vi "EditSettings.vi"(11 "Template in":string) -> (1 "Settings out":T1={"Name of test"="", "Date"=timestamp(0 s since 1904-01-01), "Location"="", "Template"="", "Soundcard"="", "resolution"=32, "Sampling rate"=48000, "Ch1 Gain "=25.0, "Ch2 Gain"=10.0, "Sample time (s)"=0.3, "Pre-trigger (s)"=0.01, "Hammer Threshold"=10.0, "Positions"=12, "Taps/Position"=5, "Set Names"="", "Freq resolution"=10.0, "Hammer cutoff"=0.0, "Mic cutoff"=0.0, "Double bounce "=0.0, "Hammer Cal"=1.0, "dB Offset"=0.0, "Accel Cal"=1.0, "Vibrometer Cal"=1.0, "Mic Cal"=1.0, "Output"=2, "Voltage Cal"=1.0, "Vibrometer Port"="ASRL27::INSTR", "Range"=50, "High Pass"=2, "Bandwidth"=25, "X Range"=[], "Y Range"=[], "dB Spread"=0.0, "Trigger"=0, "Ch_1"=1, "Ch_2"=2, "flip?"=FALSE, "60Hz"=FALSE, "Time offset"=0.0, "Piezo Cal"=1.0, "Default Notes"="", "Tom"=FALSE} {"Ch_2" min=1 step=1; "Ch_1" min=1 max=100 step=1; "Trigger" items=["Hammer (force)", "Self-tap", "Spacebar"]; "Bandwidth" items=["1 kHz"=1, "5 kHz"=5, "10 kHz"=10, "25 kHz"=25, "50 kHz"=50, "100 kHz"=100]; "High Pass" items=["Off", "13 Hz", "104 Hz"]; "Range" items=["10 mm/s"=1, "20 mm/s"=2, "50 mm/s"=5, "100 mm/s"=10, "200 mm/s"=20, "500 mm/s"=50, "1 m/s"=100, "2 m/s"=200]; "Output" items=["Accelerometer", "Speed (from acceleration)", "Microphone", "Vibrometer", "Piezo"]; "Voltage Cal" format="%#_13g"; "Ch2 Gain" format="%#_13g"; "Ch1 Gain" format="%#_13g"; "Double bounce" min=0.0; "Mic cutoff" min=0.0 format="%#_4g"; "Hammer cutoff" min=0.0 format="%#_4g"; "Freq resolution" min=0.0; "Pre-trigger (s)" format="%#_13g"; "Date" format="%<%H:%M\n%d/%m/%y>T"; "resolution" items=["16 bit"=16, "24 bit"=24, "32 bit"=32]; "Sampling rate" items=["22050 samp/s"=22050, "44100 samp/s"=44100, "48000 samp/s"=48000]}, 3 "Template out":string)   [LabVIEW 2022 SP3]
uses:
  Mic/Mic_Global.vi
  PreferencesControl.ctl
panel:
  in  "Import Cal":bool
  in  "Advanced":bool
  out "Hammer Spectrum":cluster{dbl, "df":dbl, "FFT {X}":dbl[]}[](graph)=[{0.0, "df"=1.0, "FFT {X}"=array[24000 elements]}, {0.0, "df"=40000.0, "FFT {X}"=[-20.0, -20.0]}]
  in  "Vibrometer":bool
  in  "delete":bool
  in  "Update":bool
  in  "Template":u16(ring) items=["Admittance H modified", "Admittance H", "Admittance Scratchpad", "JC H 12 radiation", "JC H 7 radiation modified modified", "JC H 7 radiation modified", "JC H 7 radiation", "JC HV 24 radiation", "Radiation ScratchPad", "ScratchPad", "TapTones ScratchPad", "TEST modified", "TEST"]
  in  "Graph Ranges":T2={"Ranges"=[{"XMin"=200.0, "XMax"=10000.0, "XInc"=2500.0, "XMinor"=500.0, "YMin"=-25.0, "YMax"=0.0, "YInc"=5.0, "YMinor"=1.0}, {"XMin"=0.0, "XMax"=0.05, "XInc"=0.025, "XMinor"=0.0025, "YMin"=-0.1, "YMax"=0.1, "YInc"=0.05, "YMinor"=0.01}, {"XMin"=0.0, "XMax"=0.3, "XInc"=0.1, "XMinor"=0.01, "YMin"=-0.1, "YMax"=0.1, "YInc"=0.05, "YMinor"=0.01}, {"XMin"=200.0, "XMax"=10000.0, "XInc"=10.0, "XMinor"=100.0, "YMin"=-30.0, "YMax"=30.0, "YInc"=5.0, "YMinor"=1.0}]}
  in  "Save":bool
  in  "Cancel Button":bool
  in  "Save as a Template":bool
  in  "Import Template":bool
  out "Template file":string
  in  "Settings":T3={"Name of test"="ScratchPad", "Date"=timestamp(0 s since 1904-01-01), "Location"="Home", "Default Template"="", "Soundcard"="OCTA-CAPTURE", "resolution"=32, "Sampling rate"=48000, "Ch1 Gain "=10.0, "Ch2 Gain"=20.0, "Sample time (s)"=0.3, "Pre-trigger (s)"=0.001, "Hammer Threshold"=0.01, "Positions"=12, "Taps/Position"=5, "Set Names"="H,V", "Freq resolution"=1.0, "Hammer cutoff"=0.025, "Mic cutoff"=0.25, "Double bounce "=0.01, "Hammer Cal"=1.0, "dB Offset"=0.0, "Accel Cal"=1.0, "Vibrometer Cal"=1.0, "Mic Cal"=49.38, "Output"=2, "Voltage Cal"=13.8, "Vibrometer Port"="ASRL27::INSTR", "Range"=50, "High Pass"=2, "Bandwidth"=25, "X Range"=[{"Minimum"=200.0, "Maximum"=10000.0, "Increment"=2500.0, "Minor Increment"=500.0, "Start"=2500.0}, {"Minimum"=0.0, "Maximum"=0.05, "Increment"=0.025, "Minor Increment"=0.0025, "Start"=0.0}, {"Minimum"=0.0, "Maximum"=0.3, "Increment"=0.1, "Minor Increment"=0.01, "Start"=0.0}, {"Minimum"=200.0, "Maximum"=10000.0, "Increment"=10.0, "Minor Increment"=100.0, "Start"=1000.0}], "Y Range"=[{"Minimum"=-25.0, "Maximum"=0.0, "Increment"=5.0, "Minor Increment"=1.0, "Start"=-25.0}, {"Minimum"=-0.1, "Maximum"=0.1, "Increment"=0.05, "Minor Increment"=0.01, "Start"=-0.1}, {"Minimum"=-0.1, "Maximum"=0.1, "Increment"=0.05, "Minor Increment"=0.01, "Start"=-0.1}, {"Minimum"=-30.0, "Maximum"=30.0, "Increment"=5.0, "Minor Increment"=1.0, "Start"=-30.0}], "dB Spread"=40.0, "Trigger"=0, "Ch_1"=1, "Ch_2"=2, "flip?"=FALSE, "60Hz"=FALSE, "Time Offset"=1.0, "Piezo Cal"=1.0, "Default Notes for template"="H,V", "Tom"=FALSE} {"Voltage Cal" format="%#_13g"; "Freq resolution" min=0.0; "Pre-trigger (s)" format="%#_13g"; "resolution" items=["16 bit"=16, "24 bit"=24, "32 bit"=32]; "Sampling rate" items=["22050 samp/s"=22050, "44100 samp/s"=44100, "48000 samp/s"=48000]; "Ch_2" min=1 step=1; "Ch_1" min=1 max=100 step=1; "Trigger" items=["Hammer (force)", "Self-tap", "Spacebar"]; "Bandwidth" items=["1 kHz"=1, "5 kHz"=5, "10 kHz"=10, "25 kHz"=25, "50 kHz"=50, "100 kHz"=100]; "High Pass" items=["Off", "13 Hz", "104 Hz"]; "Range" items=["10 mm/s"=1, "20 mm/s"=2, "50 mm/s"=5, "100 mm/s"=10, "200 mm/s"=20, "500 mm/s"=50, "1 m/s"=100, "2 m/s"=200]; "Output" items=["Accelerometer", "Speed (accelerometer)", "Microphone", "Vibrometer"]; "Ch2 Gain" format="%#_13g"; "Ch1 Gain" format="%#_13g"; "Double bounce" min=0.0; "Mic cutoff" min=0.0 format="%#_4g"; "Hammer cutoff" min=0.0 format="%#_4g"; "Date" format="%<%H:%M\n%d/%m/%y>T"}
  out "Hammer Data":cluster{dbl, "dt":dbl, "Y":dbl[]}[](graph)=[{0.0, "dt"=2.0833333333333333e-05, "Y"=array[14400 elements]}, {0.0, "dt"=0.0, "Y"=[]}]
  out "Microphone Data":cluster{dbl, "dt":dbl, "Y":dbl[]}[](graph)=[{0.0, "dt"=2.0833333333333333e-05, "Y"=array[14400 elements]}, {0.0, "dt"=0.0, "Y"=[]}]
  out "Average FRF":cluster{dbl, "df":dbl, dbl[]}[](graph)=[{0.0, "df"=1.0, array[24000 elements]}, {0.0, "df"=1.0, array[24000 elements]}]
  # "Adjust default scale ranges"
  # "Hz"
  # "dB"
  # "dB"
  # "sec"
  # "sec"
  # "mV/Pa"
  # "mV/m/s2"
  # "mV/mm/s"
  # "V/N"
  # "sec"
  # "sec"
  # "mV/N"
  # "a.u."
  # "a.u."
  # "sec"
  # "X Min      X Max      X Inc        X Minor   Y Min      Y Max       Y Inc        Y Minor"
  # "Hammer Spectrum\n\nHammer Level Meter \n\nMic Level Meter\n\nFreq Response Plot"
  # "mV/Pa"
  # "mV/m/s2"
  # "mV/mm/s"
  # "Hz"
  # "V/N"
  # "dB"
  # "sec"
  # "sec"
  # "dB"
  # "mV/N"
  # "a.u."
  # "sec"
  # "a.u."
  # "sec"
  # "sec"
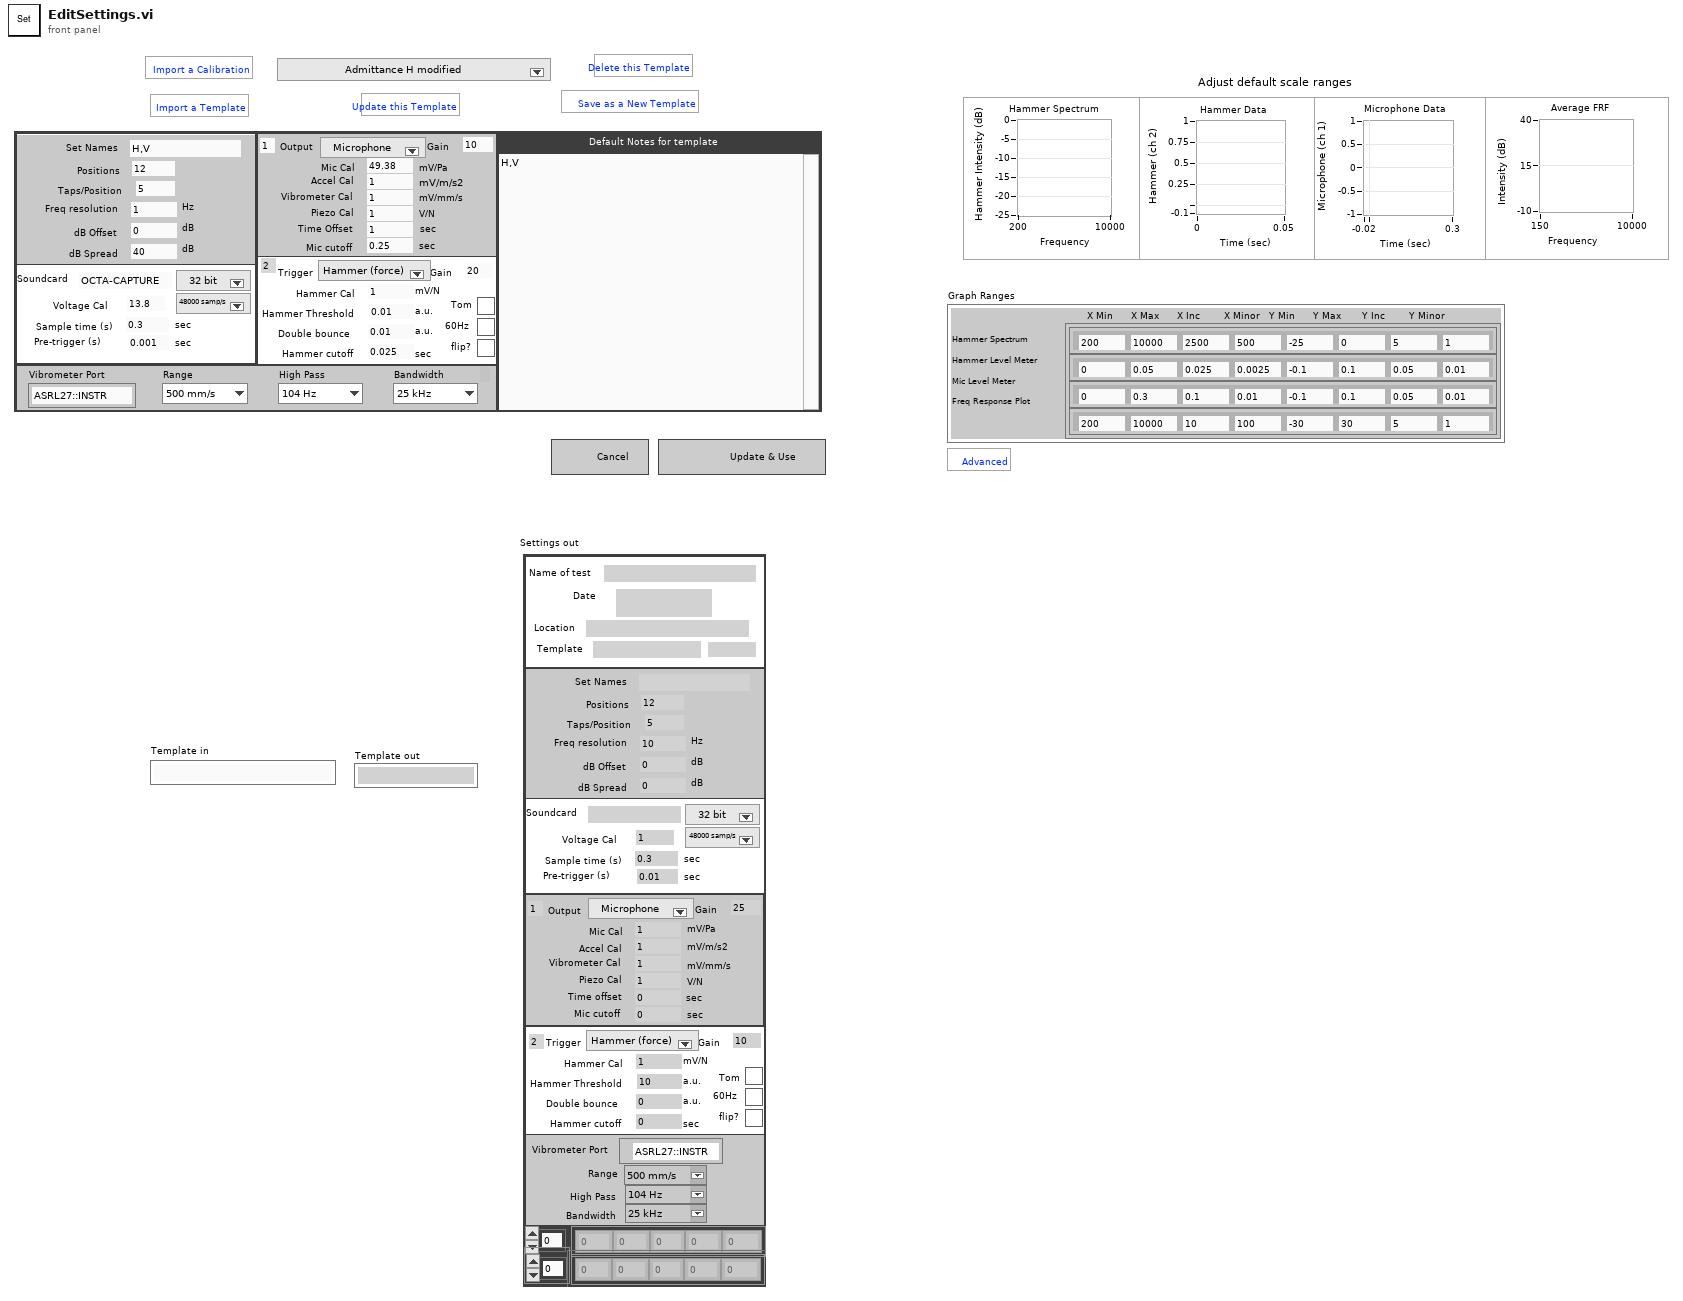
[diagram p1: front panel]
types:
  T1 = typedef "PreferencesControl.ctl" = cluster{"Name of test":string, "Date":timestamp, "Location":string, "Template":string, "Soundcard":string, "resolution":u16, "Sampling rate":u16, "Ch1 Gain ":dbl, "Ch2 Gain":dbl, "Sample time (s)":dbl, "Pre-trigger (s)":dbl, "Hammer Threshold":dbl, "Positions":i16, "Taps/Position":i16, "Set Names":string, "Freq resolution":dbl, "Hammer cutoff":dbl, "Mic cutoff":dbl, "Double bounce ":dbl, "Hammer Cal":dbl, "dB Offset":dbl, "Accel Cal":dbl, "Vibrometer Cal":dbl, "Mic Cal":dbl, "Output":u16, "Voltage Cal":dbl, "Vibrometer Port":refnum<visa-resource-name>, "Range":u16, "High Pass":u16, "Bandwidth":u16, "X Range":cluster{"Minimum":dbl, "Maximum":dbl, "Increment":dbl, "Minor Increment":dbl, "Start":dbl}[], "Y Range":cluster{"Minimum":dbl, "Maximum":dbl, "Increment":dbl, "Minor Increment":dbl, "Start":dbl}[], "dB Spread":dbl, "Trigger":u16, "Ch_1":u8, "Ch_2":u8, "flip?":bool, "60Hz":bool, "Time offset":dbl, "Piezo Cal":dbl, "Default Notes":string, "Tom":bool}
  T2 = cluster{"Ranges":cluster{"XMin":dbl, "XMax":dbl, "XInc":dbl, "XMinor":dbl, "YMin":dbl, "YMax":dbl, "YInc":dbl, "YMinor":dbl}[]}
  T3 = cluster{"Name of test":string, "Date":timestamp, "Location":string, "Default Template":string, "Soundcard":string, "resolution":u16, "Sampling rate":u16, "Ch1 Gain ":dbl, "Ch2 Gain":dbl, "Sample time (s)":dbl, "Pre-trigger (s)":dbl, "Hammer Threshold":dbl, "Positions":i16, "Taps/Position":i16, "Set Names":string, "Freq resolution":dbl, "Hammer cutoff":dbl, "Mic cutoff":dbl, "Double bounce ":dbl, "Hammer Cal":dbl, "dB Offset":dbl, "Accel Cal":dbl, "Vibrometer Cal":dbl, "Mic Cal":dbl, "Output":u16, "Voltage Cal":dbl, "Vibrometer Port":string, "Range":u16, "High Pass":u16, "Bandwidth":u16, "X Range":cluster{"Minimum":dbl, "Maximum":dbl, "Increment":dbl, "Minor Increment":dbl, "Start":dbl}[], "Y Range":cluster{"Minimum":dbl, "Maximum":dbl, "Increment":dbl, "Minor Increment":dbl, "Start":dbl}[], "dB Spread":dbl, "Trigger":u16, "Ch_1":u8, "Ch_2":u8, "flip?":bool, "60Hz":bool, "Time Offset":dbl, "Piezo Cal":dbl, "Default Notes for template":string, "Tom":bool}
  T4 = enum8{"Enabled", "Disabled", "Disabled and Grayed Out"}
  T5 = enum32{"Invalid", "Default", "Floating", "Floating/Auto-Hide", "Modal"}
  T6 = typedef "LVRangeTypeDef.ctl" = cluster{"Minimum":dbl, "Maximum":dbl, "Increment":dbl, "Minor Increment":dbl, "Start":dbl}
  T7 = typedef "LVRectTypeDef.ctl" = cluster{"Left":i16, "Top":i16, "Right":i16, "Bottom":i16}
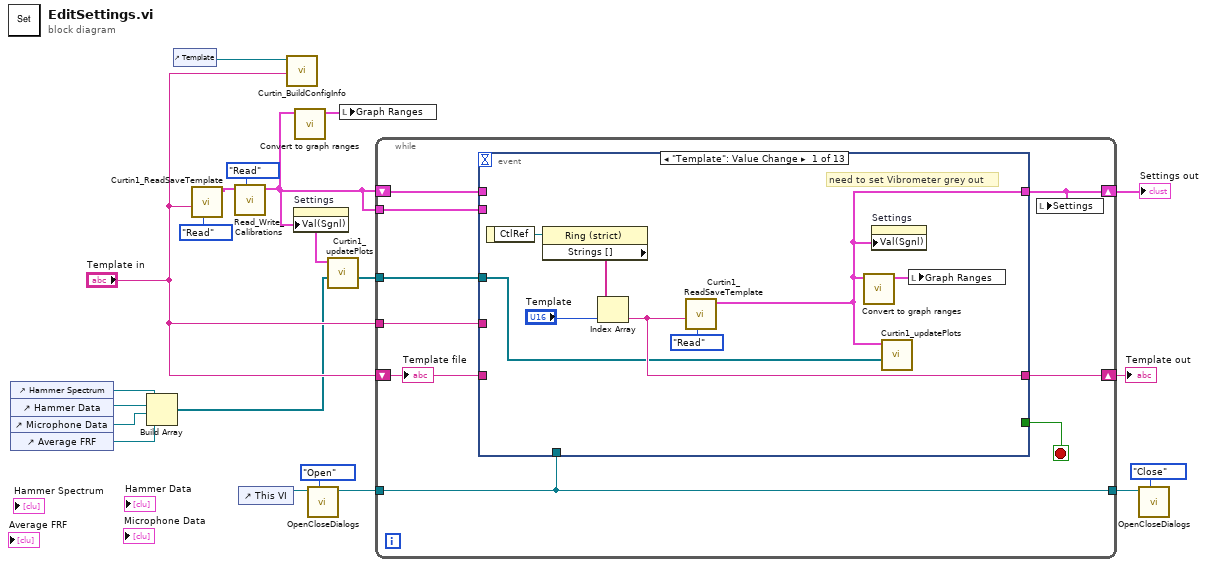
[diagram p0: block diagram]
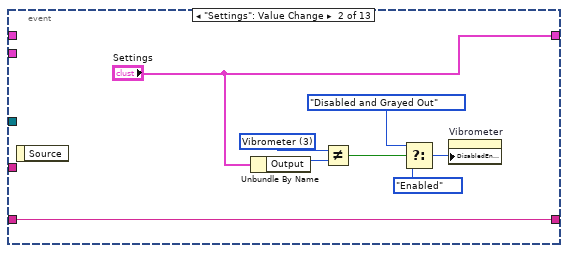
[diagram p2: hidden frame]
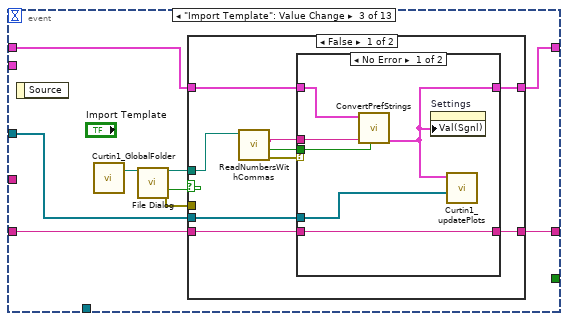
[diagram p3: hidden frame]
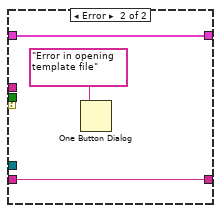
[diagram p4: hidden frame]
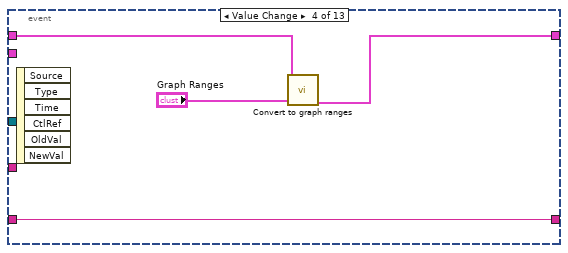
[diagram p6: hidden frame]
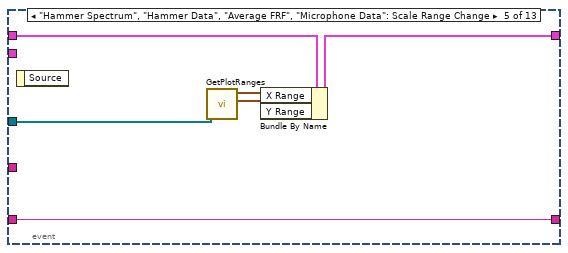
[diagram p7: hidden frame]
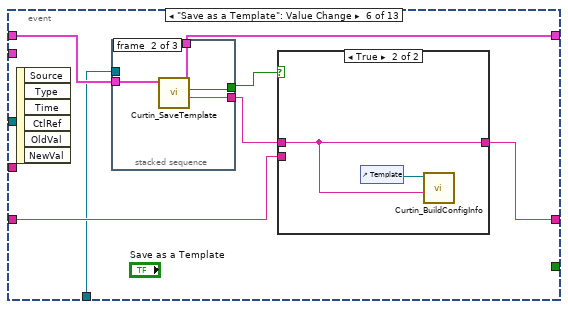
[diagram p8: hidden frame]
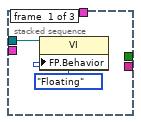
[diagram p9: hidden frame]
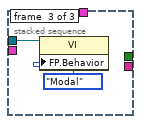
[diagram p10: hidden frame]
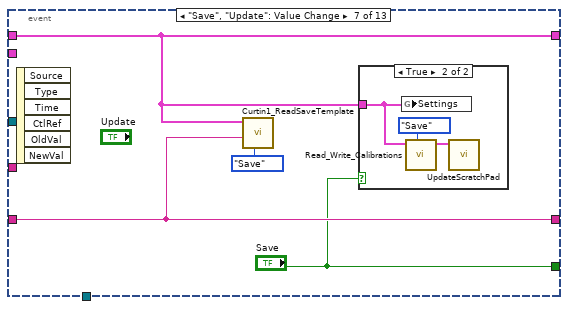
[diagram p12: hidden frame]
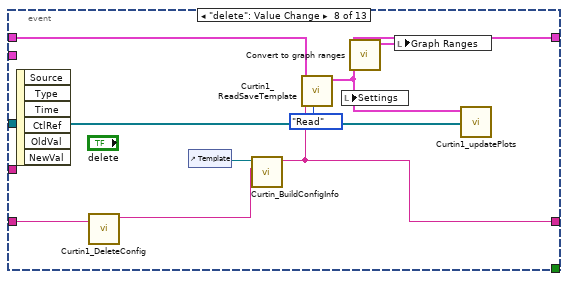
[diagram p14: hidden frame]
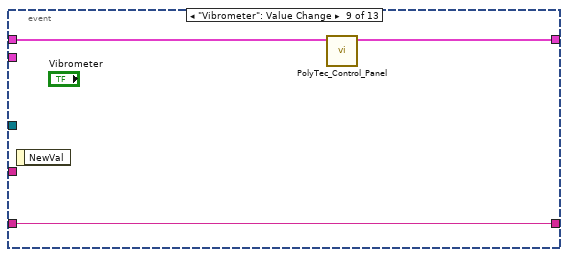
[diagram p15: hidden frame]
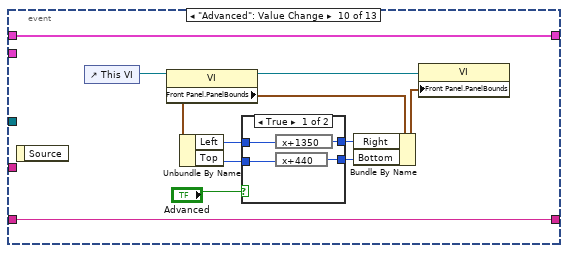
[diagram p16: hidden frame]
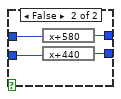
[diagram p17: hidden frame]
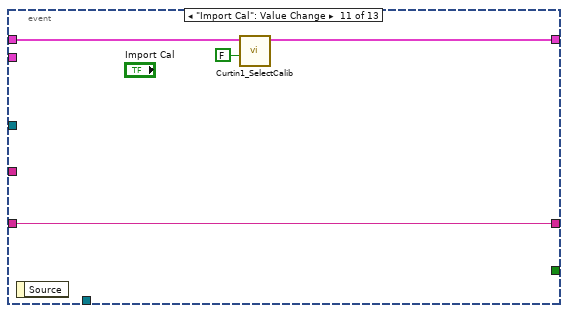
[diagram p18: hidden frame]
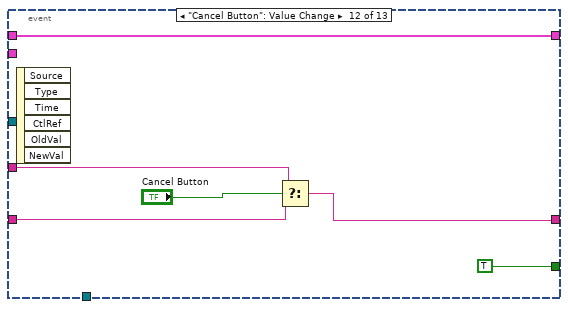
[diagram p19: hidden frame]
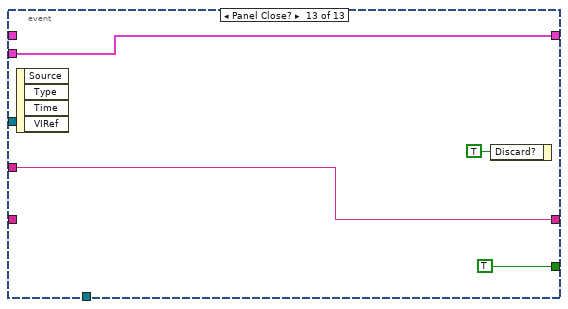
[diagram p20: hidden frame]
diagram:
  n1 = control-ref of="Hammer Spectrum"() -> (w11:refnum<vi>)
  n2 = control-ref of="Hammer Data"() -> (w12:refnum<vi>)
  n3 = control-ref of="Microphone Data"() -> (w13:refnum<vi>)
  n4 = control-ref of="Average FRF"() -> (w14:refnum<vi>)
  n5 = Build Array(w11, w12, w13, w14) -> (w10:refnum<vi>[])
  n6 = control-ref of="Template"() -> (w16:refnum<vi>)
  n7 = call "Curtin1_ReadSaveTemplate.vi"("Task"=enum16{"Save", "Read", "List"}."Read", "Template"="Template in") -> ("Settings out"=w7:T1)  [unwired: 6 in, 3 out]
  n8 = call "Read_Write_Calibrations.vi"("Task"=enum16{"Save", "Read", "List"}."Read", "Settings in"=w7) -> ("Settings out"=w6:T1)  [unwired: 7 in, 2 out]
  n9 = control-ref of="This VI"() -> (w4:refnum<vi>)
  n10 = call "Curtin_BuildConfigInfo.vi"("Test Template in"="Template in", "ComboBox in"=w16) -> ()  [unwired: 8 in, 2 out]
  n11 = property on="Settings" class="Clust (strict)"("Val(Sgnl)"=w6) -> ()  [unwired: 2 in, 2 out]
  n12 = call "Convert to graph ranges.vi"("Settings in"=w6) -> ("Graph Ranges out"=w17:T2)  [unwired: 9 in, 1 out]
  n13 = call "OpenCloseDialogs.vi"("Task"=enum16{"Open", "Close"}."Open", "VI in"=w4) -> ("VI out"=w1:refnum<vi>)  [unwired: 8 in, 1 out]
  n14 = call "Curtin1_updatePlots.vi"("plots"=w10, "Settings"=w6) -> ()  [unwired: 10 in]
  n15 = local write "Graph Ranges"(w17) -> ()
  n16 = while {
    shift-right: [w23] -> w9
    shift-left: w6 -> [w27]
    shift-right: [w26] -> w18
    shift-left: "Template in" -> [w25]
    tunnel: "Template in" -> [w24]
    tunnel: w6 -> [w22]
    tunnel: w10 -> [w21]
    tunnel: [w20] -> w2
    tunnel: w1 -> [w20]
    stop <- w28 stop-if-true
    n17 = event shown="[0] \"Template\": Value Change" {
      selector: _ -> [_ _ _ _ _ _ _ _ _ _ _ _ _]
      dyn-events: _ -> [_ _ _ _ _ _ _ _ _ _ _ _ _]
      timeout: _ -> [_ _ _ _ _ _ _ _ _ _ _ _ _]
      tunnel: [_ _ _ _ _ _ "Save" _ _ _ _ TRUE TRUE] -> w28
      tunnel: w27 -> [_ _ w51 w75 w80 w88 w102 w113 w119 w131 w142 w148 _]
      tunnel: [w29 "Settings" w50 w74 w79 w86 w102 w109 w118 w131 w141 w148 w150] -> w23
      tunnel: [w31 w44 w49 w77 w78 w90 w104 w112 w120 w121 w143 w144 w151] -> w26
      tunnel: w25 -> [_ w44 w48 w77 w78 w89 w104 w117 w120 w121 w143 w145 _]
      tunnel: w24 -> [_ _ _ _ _ _ _ _ _ _ _ w146 w151]
      tunnel: w22 -> [_ _ _ _ _ _ _ _ _ _ _ _ w150]
      tunnel: w21 -> [w30 _ w45 _ w81 _ _ w110 _ _ _ _ _]
      tunnel: w20 -> [_ _ _ _ _ w85 _ _ _ _ _ _ _]
      event "Template": Value Change {
        # "need to set Vibrometer grey out"
        n18 = event-data() -> ("CtlRef"=w34:refnum<vi>)  [unwired: 1 in]
        n19 = property class="Ring (strict)"(reference=w34) -> ("Strings []"=w33:string[])  [unwired: 1 in, 2 out]
        n20 = Index Array(array=w33, index="Template") -> (element=w31:string)
        n21 = call "Curtin1_ReadSaveTemplate.vi"("Task"=enum16{"Save", "Read", "List"}."Read", "Template"=w31) -> ("Settings out"=w29:T1)  [unwired: 6 in, 3 out]
        n22 = call "Convert to graph ranges.vi"("Settings in"=w29) -> ("Graph Ranges out"=w36:T2)  [unwired: 9 in, 1 out]
        n23 = property on="Settings" class="Clust (strict)"("Val(Sgnl)"=w29) -> ()  [unwired: 2 in, 2 out]
        n24 = call "Curtin1_updatePlots.vi"("plots"=w30, "Settings"=w29) -> ()  [unwired: 10 in]
        n25 = local write "Graph Ranges"(w36) -> ()
      }
      event "Settings": Value Change {
        w39 = u16 3 items=["Acclerometer", "Displacement", "Microphone", "Vibrometer"] ("Output")
        n26 = event-data() -> ()  [unwired: 1 in, 1 out]
        n27 = Unbundle By Name("Settings") -> ("Output"=w38:u16)
        n28 = Not Equal?(x=w39, y=w38) -> (x != y?=w40:bool)
        n29 = Select(t=T4."Disabled and Grayed Out" ("Disabled"), s=w40, f=T4."Enabled" ("Disabled")) -> (s? t:f=w43:T4)
        n30 = property on="Vibrometer" class="Bool"("DisabledEnum"=w43) -> ()  [unwired: 2 in, 2 out]
      }
      event "Import Template": Value Change {
        n31 = event-data() -> ()  [unwired: 1 in, 1 out]
        n32 = call "Curtin1_GlobalFolder.vi"() -> ("LabVIEW Data Path"=w46:path)  [unwired: 1 in, 1 out]
        n33 = call "File Dialog"("start path"=w46) -> ("selected path"=w53:path, "cancelled"=w52:bool, "error out"=w47:errorcluster)  [unwired: 11 in, 1 out]
        n34 = case shown="False" w52 {
          tunnel: w53 -> [w57 _]
          tunnel: w51 -> [w62 w73]
          tunnel: [w61 w73] -> w50
          tunnel: [w60 w72] -> w49
          tunnel: w48 -> [w59 w72]
          tunnel: w47 -> [_ _]
          tunnel: w45 -> [w58 _]
          frame False {
            n35 = call "ReadNumbersWithCommas.vi"("file (use dialog)"=w57) -> ("error out"=w55:errorcluster, "comma?"=w54:bool, "text"=w56:string)  [unwired: 7 in, 1 out]
            n36 = case shown="No Error" w55 {
              tunnel: w62 -> [w66 w71]
              tunnel: [w64 w71] -> w61
              tunnel: [w68 w69] -> w60
              tunnel: w59 -> [w68 w69]
              tunnel: w56 -> [w67 _]
              tunnel: w58 -> [w65 _]
              tunnel: w54 -> [w63 _]
              frame No Error {
                n37 = call "ConvertPrefStrings.vi"("Comma?"=w63, "String In"=w67, "Settings"=w66) -> ("Settings"=w64:T1)  [unwired: 7 in, 1 out]
                n38 = property on="Settings" class="Clust (strict)"("Val(Sgnl)"=w64) -> ()  [unwired: 2 in, 2 out]
                n39 = call "Curtin1_updatePlots.vi"("plots"=w65, "Settings"=w64) -> ()  [unwired: 10 in]
              }
              frame Error {
                n40 = One Button Dialog(message="Error in opening template file") -> ()  [unwired: 1 in, 1 out]
              }
            }
          }
          frame True {
          }
        }
      }
      event "Graph Ranges.Ranges": Value Change {
        n41 = event-data() -> ()  [unwired: 1 in, 6 out]
        n42 = call "Convert to graph ranges.vi"("Graph Ranges in"="Graph Ranges", "Settings in"=w75) -> ("Settings out"=w74:T1)  [unwired: 8 in, 1 out]
      }
      event "Hammer Spectrum", "Hammer Data", "Average FRF", "Microphone Data": Scale Range Change {
        n43 = event-data() -> ()  [unwired: 1 in, 1 out]
        n44 = call "GetPlotRanges.vi"("plots"=w81) -> ("Yscales"=w83:T6[], "Xscales"=w82:T6[])  [unwired: 9 in]
        n45 = Bundle By Name(cluster=w80, "X Range"=w82, "Y Range"=w83) -> (w79:T1)
      }
      event "Save as a Template": Value Change {
        n46 = event-data() -> ()  [unwired: 1 in, 6 out]
        n47 = stacked-sequence {
          tunnel: w85 -> [w92 _ w98]
          tunnel: w88 -> [_ w96 _]
          tunnel: [_ w95 _] -> w87
          tunnel: [_ w94 _] -> w84
          tunnel: [_ w93 _] -> w86
          frame #0 {
            n48 = property class="VI"(reference=w92, "FP.Behavior"=T5."Floating" ("Front Panel Window:Behavior")) -> ()  [unwired: 1 in, 2 out]
          }
          frame #1 {
            n49 = call "Curtin_SaveTemplate.vi"("Settings in"=w96) -> ("New Template"=w95:string, "Good?"=w94:bool, "Settings out"=w93:T1)  [unwired: 8 in]
          }
          frame #2 {
            n50 = property class="VI"(reference=w98, "FP.Behavior"=T5."Modal" ("Front Panel Window:Behavior")) -> ()  [unwired: 1 in, 2 out]
          }
        }
        n51 = case shown="True" w84 {
          tunnel: w87 -> [_ w100]
          tunnel: [w99 w100] -> w90
          tunnel: w89 -> [w99 _]
          frame False {
          }
          frame True {
            n52 = control-ref of="Template"() -> (w101:refnum<vi>)
            n53 = call "Curtin_BuildConfigInfo.vi"("Test Template in"=w100, "ComboBox in"=w101) -> ()  [unwired: 8 in, 2 out]
          }
        }
      }
      event "Save", "Update": Value Change {
        n54 = event-data() -> ()  [unwired: 1 in, 6 out]
        n55 = call "Curtin1_ReadSaveTemplate.vi"("Task"=enum16{"Save", "Read", "List"}."Save", "Template"=w104, "Settings"=w102) -> ()  [unwired: 5 in, 4 out]
        n56 = case shown="True" "Save" {
          tunnel: w102 -> [_ w107]
          frame False {
          }
          frame True {
            n57 = global write "Mic_Global.vi" "Settings"(w107) -> ()
            n58 = call "Read_Write_Calibrations.vi"("Task"=enum16{"Save", "Read", "List"}."Save", "Settings in"=w107) -> ("Settings out"=w106:T1)  [unwired: 7 in, 2 out]
            n59 = call "UpdateScratchPad.vi"("Settings"=w106) -> ()  [unwired: 9 in, 2 out]
          }
        }
      }
      event "delete": Value Change {
        n60 = event-data() -> ()  [unwired: 1 in, 6 out]
        n61 = call "Curtin1_DeleteConfig.vi"("Test Configuration"=w117) -> ("New File"=w111:string)  [unwired: 10 in]
        n62 = control-ref of="Template"() -> (w116:refnum<vi>)
        n63 = call "Curtin_BuildConfigInfo.vi"("Test Template in"=w111, "ComboBox in"=w116) -> ("template"=w112:string)  [unwired: 8 in, 1 out]
        n64 = call "Curtin1_ReadSaveTemplate.vi"("Task"=enum16{"Save", "Read", "List"}."Read", "Template"=w112, "Settings"=w113) -> ("Settings out"=w109:T1)  [unwired: 5 in, 3 out]
        n65 = local write "Settings"(w109) -> ()
        n66 = call "Convert to graph ranges.vi"("Settings in"=w109) -> ("Graph Ranges out"=w115:T2)  [unwired: 9 in, 1 out]
        n67 = local write "Graph Ranges"(w115) -> ()
        n68 = call "Curtin1_updatePlots.vi"("plots"=w110, "Settings"=w109) -> ()  [unwired: 10 in]
      }
      event "Vibrometer": Value Change {
        n69 = event-data() -> ()  [unwired: 1 in, 1 out]
        n70 = call "PolyTec_Control_Panel.vi"("Settings in"=w119) -> ("Settings Out"=w118:T1)  [unwired: 8 in, 2 out]
      }
      event "Advanced": Value Change {
        n71 = event-data() -> ()  [unwired: 1 in, 1 out]
        n72 = control-ref of="This VI"() -> (w123:refnum<vi>)
        n73 = property class="VI"(reference=w123) -> (reference out=w129:refnum<vi>, "Front Panel.PanelBounds"=w124:T7)  [unwired: 1 in, 1 out]
        n74 = Unbundle By Name(w124) -> ("Left"=w125:i16, "Top"=w127:i16)
        n75 = case shown="True" "Advanced" {
          tunnel: [w135 w139] -> w128
          tunnel: w127 -> [w134 w138]
          tunnel: [w133 w137] -> w126
          tunnel: w125 -> [w132 w136]
          frame True {
            n76 = expression code="x+1350"(w132) -> (w133:i16)
            n77 = expression code="x+440"(w134) -> (w135:i16)
          }
          frame False {
            n78 = expression code="x+580"(w136) -> (w137:i16)
            n79 = expression code="x+440"(w138) -> (w139:i16)
          }
        }
        n80 = Bundle By Name(cluster=w124, "Right"=w126, "Bottom"=w128) -> (w130:T7)
        n81 = property class="VI"(reference=w129, "Front Panel.PanelBounds"=w130) -> ()  [unwired: 1 in, 2 out]
      }
      event "Import Cal": Value Change {
        n82 = event-data() -> ()  [unwired: 1 in, 1 out]
        n83 = call "Curtin1_SelectCalib.vi"("Save?"=FALSE ("goal"), "Settings in"=w142) -> ("Settings out"=w141:T1)  [unwired: 9 in]
      }
      event "Cancel Button": Value Change {
        n84 = event-data() -> ()  [unwired: 1 in, 6 out]
        n85 = Select(t=w146, s="Cancel Button", f=w145) -> (s? t:f=w144:string)
      }
      event Panel Close? {
        n86 = event-data() -> ()  [unwired: 1 in, 4 out]
        n87 = event-data("Discard?"=TRUE) -> ()  [unwired: 1 in, 1 out]
      }
    }
    n88 = local write "Settings"(w23) -> ()
    "Template file" <- w25
  }
  "Template out" <- w18
  "Settings out" <- w9
  n89 = call "OpenCloseDialogs.vi"("Task"=enum16{"Open", "Close"}."Close", "VI in"=w2) -> ()  [unwired: 8 in, 2 out]
